vi "SOUR_POW_MODE.vi"(0 "VISA IN":refnum<visa-resource-name>, 2 "Source State":string(combo), 5 "error in":errorcluster, 7 "Channel":i32, 9 "Port number":i32, 11 "Source":string) -> (14 "VISA Out":refnum<visa-resource-name>, 19 "error out":errorcluster)   [LabVIEW 2018, in "PNA-X.lvlib"]
doc: "SOURce<cnum>:POWer<port>:MODE <state>, [src] \n1830\n\n(Read-Write) Sets the state of PNA source for the specified port. \nLearn more about the PNA internal second source \nParameters \n<cnum> Any existing channel number. If unspecified, value is set to 1 \n<port> Port number of the PNA. If unspecified, <port> is set to 1. To make settings for \nports that are not simple numbers, use the [src] argument. \n<state> Source state. Choose from: \nAUTO Source power is turned ON when required for a measurement. \nON Source power is always ON regardless of the measurement. \nOFF Source power is always OFF regardless of the measurement. \nNote: ON and OFF are valid only on PNA models with two sources. \n[src] String. (NOT case sensitive). Source port. Optional. Use SOUR:CAT? to \nreturn a list of valid port names. \nWhile this argument can be used to make settings for ALL ports, it is designed \nto access ports that are not simple numbers, such as \"Port 1 Src2\". Otherwise, \nthe <port> argument performs the same function. If both arguments are \nspecified, [src] takes priority. \nExamples SOUR:POW:MODE ON \nsource2:power4:mode OFF \nsour:pow:mode 1, \"Port 1 Src2\" \nQuery Syntax SOURce<cnum>:POWer<port>:MODE? [src} \nReturn Type Character \nDefault Auto"
uses:
  PNA-X.lvlib
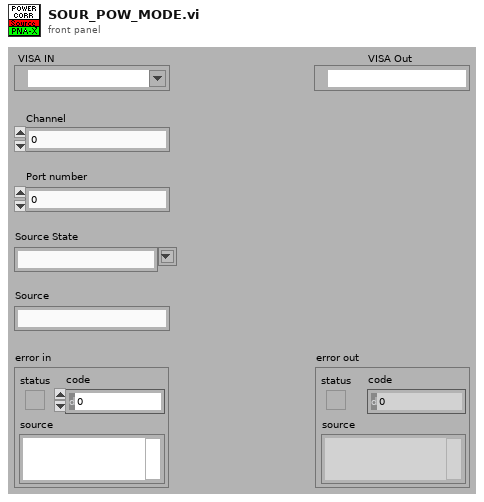
[diagram p1: front panel]
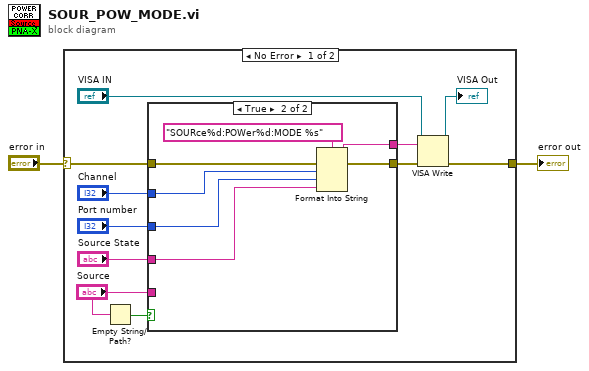
[diagram p0: block diagram]
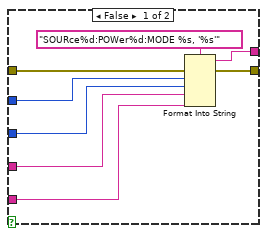
[diagram p2: hidden frame]
diagram:
  n1 = case shown="No Error" "error in" {
    selector: "error in" -> [w13 w29]
    tunnel: [w9 w29] -> w1
    frame No Error {
      n2 = Empty String/Path?(string/path="Source") -> (empty?=w4:bool)
      n3 = case shown="True" w4 {
        tunnel: w13 -> [w17 w28]
        tunnel: [w16 w27] -> w12
        tunnel: [w15 w26] -> w11
        tunnel: "Channel" -> [w18 w24]
        tunnel: "Port number" -> [w19 w23]
        tunnel: "Source State" -> [w20 w22]
        tunnel: "Source" -> [w14 _]
        frame False {
          n4 = Format Into String(format string="SOURce%d:POWer%d:MODE %s, '%s'" ("Cmdline"), error in=w17, w18, w19, w20, w14) -> (resulting string=w15:string, error out=w16:errorcluster)  [unwired: 1 in]
        }
        frame True {
          n5 = Format Into String(format string="SOURce%d:POWer%d:MODE %s" ("Cmdline"), error in=w28, w24, w23, w22) -> (resulting string=w26:string, error out=w27:errorcluster)  [unwired: 1 in]
        }
      }
      n6 = VISA Write(VISA resource name="VISA IN", write buffer=w11, error in (no error)=w12) -> (VISA resource name out=→"VISA Out":refnum<visa-resource-name>, error out=w9:errorcluster)  [unwired: 1 out]
    }
    frame Error {
    }
  }
  "error out" <- w1
